vi "Configure Hardware.vi"(8 "error in (no error)":errorcluster, 11 "HW Resources In":T1={"Data Source"=0, "Counter Configuration"={"DAQmx Task"="", "Counter(s)"="Dev2/ctr0", "samples per readout"=100}, "ADC Configuration"={"DAQmx Task"="", "Channel(s)"="Dev2/ctr0", "samples per readout"=100, "Sample Rate (s/s)"=100, "Max Voltage"=100.0, "Min Voltage"=100.0}} {"Data Source" items=["Counter", "ADC"]}) -> (0 "error out":errorcluster, 3 "HW Resources Out":T1={"Data Source"=0, "Counter Configuration"={"DAQmx Task"="", "Counter(s)"="Dev2/ctr0", "samples per readout"=100}, "ADC Configuration"={"DAQmx Task"="", "Channel(s)"="Dev2/ctr0", "samples per readout"=100, "Sample Rate (s/s)"=100, "Max Voltage"=100.0, "Min Voltage"=100.0}} {"Data Source" items=["Counter", "ADC"]})   [LabVIEW 2013, in "Acquisition.lvlib"]
doc: "Configure the hardware."
uses:
  Acquisition.lvlib
  Hardware Configuration.ctl
  Counter Configuration.ctl
  ADC/ADC Configuration.ctl
  <vilib>/DAQmx/create/channels.llb/DAQmx Create Channel (CI-Period).vi
  <vilib>/DAQmx/configure/timing.llb/DAQmx Timing (Implicit).vi
  <vilib>/DAQmx/create/channels.llb/DAQmx Create Channel (AI-Voltage-Basic).vi
  <vilib>/DAQmx/configure/timing.llb/DAQmx Timing (Sample Clock).vi
  <resource>/objmgr/daqmx.rc
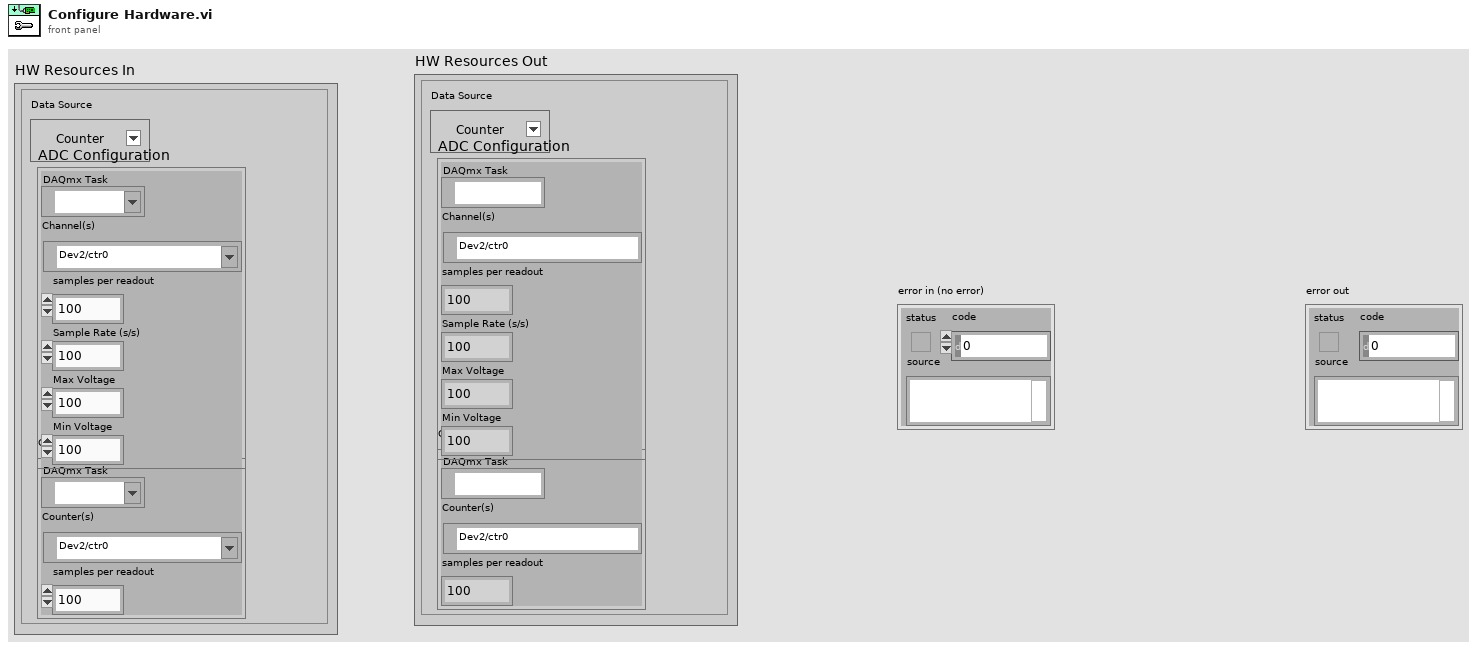
[diagram p1: front panel]
types:
  T1 = typedef "Acquisition.lvlib/Hardware Configuration.ctl" = cluster{"Data Source":u16, "Counter Configuration":T2, "ADC Configuration":T3}
  T2 = typedef "Acquisition.lvlib/Counter Configuration.ctl" = cluster{"DAQmx Task":refnum<k21>, "Counter(s)":tag, "samples per readout":i32}
  T3 = typedef "Acquisition.lvlib/ADC Configuration.ctl" = cluster{"DAQmx Task":refnum<k21>, "Channel(s)":tag, "samples per readout":i32, "Sample Rate (s/s)":i32, "Max Voltage":dbl, "Min Voltage":dbl}
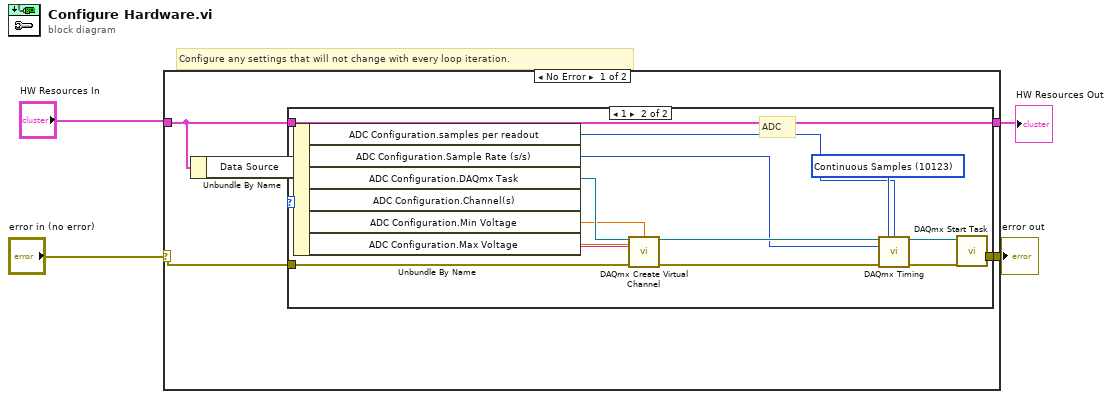
[diagram p0: block diagram]
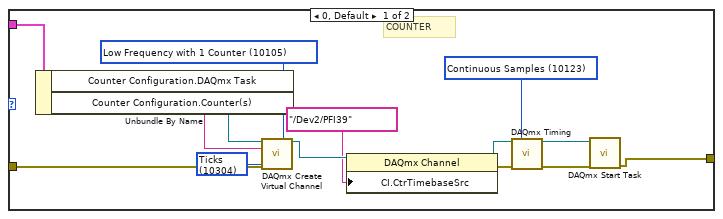
[diagram p2: hidden frame]
diagram:
  # "Configure any settings that will not change with every loop iteration."
  n1 = case shown="No Error" "error in (no error)" {
    selector: "error in (no error)" -> [w8 w37]
    tunnel: [w7 w37] -> w3
    tunnel: "HW Resources In" -> [w6 w38]
    tunnel: [w6 w38] -> w2
    frame No Error {
      n2 = Unbundle By Name(w6) -> ("Data Source"=w5:u16)
      n3 = case shown="1" w5 {
        tunnel: w8 -> [w20 w34]
        tunnel: w6 -> [w19 w33]
        tunnel: [w15 w29] -> w7
        frame 0, Default {
          w13 = 10105 items=["Low Frequency with 1 Counter"=10105, "High Frequency with 2 Counters"=10157, "Large Range with 2 Counters"=10205] ("measurement method")
          w14 = 10304 items=["Seconds"=10364, "Ticks"=10304, "From Custom Scale"=10065] ("units")
          w18 = 10123 items=["Finite Samples"=10178, "Continuous Samples"=10123, "Hardware Timed Single Point"=12522] ("sample mode")
          # "COUNTER"
          n4 = Unbundle By Name(w19) -> ("Counter Configuration.DAQmx Task"=w22:refnum<k21>, "Counter Configuration.Counter(s)"=w21:tag)
          n5 = call-poly <vilib>:"DAQmx Create Virtual Channel.vi"("task in"=w22, "measurement method"=w13, "counter"=w21, "units"=w14, "error in"=w20) -> ("task out"=w12:refnum<k21>)  [unwired: 9 in, 1 out]
          n6 = property class="DAQmx Channel"(reference=w12, "CI.CtrTimebaseSrc"=tag "/Dev2/PFI39" ("Counter Source")) -> (reference out=w11:refnum<k21>, error out=w10:errorcluster)  [unwired: 1 in]
          n7 = call-poly <vilib>:"DAQmx Timing.vi"("task/channels in"=w11, "sample mode"=w18, "error in"=w10) -> ("task out"=w16:refnum<k21>, "error out"=w17:errorcluster)  [unwired: 11 in]
          n8 = call <vilib>:"DAQmx Start Task.vi"("task/channels in"=w16, "error in"=w17) -> ("error out"=w15:errorcluster)  [unwired: 12 in, 1 out]
        }
        frame 1 {
          w32 = 10123 items=["Finite Samples"=10178, "Continuous Samples"=10123, "Hardware Timed Single Point"=12522] ("sample mode")
          # "ADC"
          n9 = Unbundle By Name(w33) -> ("ADC Configuration.samples per readout"=w23:i32, "ADC Configuration.Sample Rate (s/s)"=w24:i32, "ADC Configuration.DAQmx Task"=w36:refnum<k21>, "ADC Configuration.Channel(s)"=w35:tag, "ADC Configuration.Min Voltage"=w27:dbl, "ADC Configuration.Max Voltage"=w28:dbl)
          n10 = call-poly <vilib>:"DAQmx Create Virtual Channel.vi"("task in"=w36, "maximum value"=w28, "minimum value"=w27, "physical channels"=w35, "error in"=w34) -> ("task out"=w25:refnum<k21>, "error out"=w26:errorcluster)  [unwired: 9 in]
          n11 = call-poly <vilib>:"DAQmx Timing.vi"("task/channels in"=w25, "sample mode"=w32, "samples per channel"=w23, "rate"=w24, "error in"=w26) -> ("task out"=w30:refnum<k21>, "error out"=w31:errorcluster)  [unwired: 9 in]
          n12 = call <vilib>:"DAQmx Start Task.vi"("task/channels in"=w30, "error in"=w31) -> ("error out"=w29:errorcluster)  [unwired: 12 in, 1 out]
        }
      }
    }
    frame Error {
    }
  }
  "error out" <- w3
  "HW Resources Out" <- w2
